vi "Next.vi"(0 "object in":refnum<class "BFSTreeIterator.lvclass">, 5 "Error In":errorcluster) -> (14 "object out":refnum<class "BFSTreeIterator.lvclass">, 16 "Next":refnum<class "Element.lvclass">, 19 "Error Out":errorcluster)   [LabVIEW 2024, in "BFSTreeIterator.lvclass"]
doc: "Gets next item in the traversal order. Also prepare for upcoming nodes."
uses:
  BFSTreeIterator.lvclass
  Element_interface/Element.lvclass
  BFSTreeIterator.lvclass/BFSTreeIterator.ctl
  Node_class/Node.lvclass
  C:/Users/burakkorkmaz/Desktop/Leveling/labview-desing-patterns/Iterator Pattern/Element_interface/Element.lvclass
panel:
  # "Connector Pane"
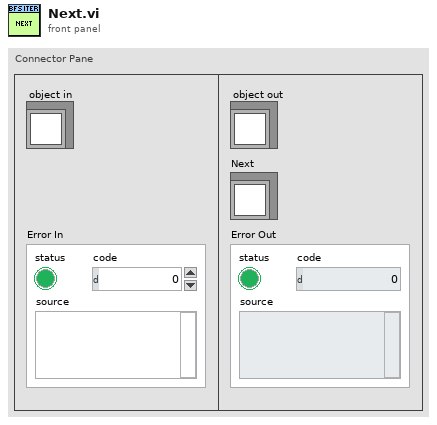
[diagram p1: front panel]
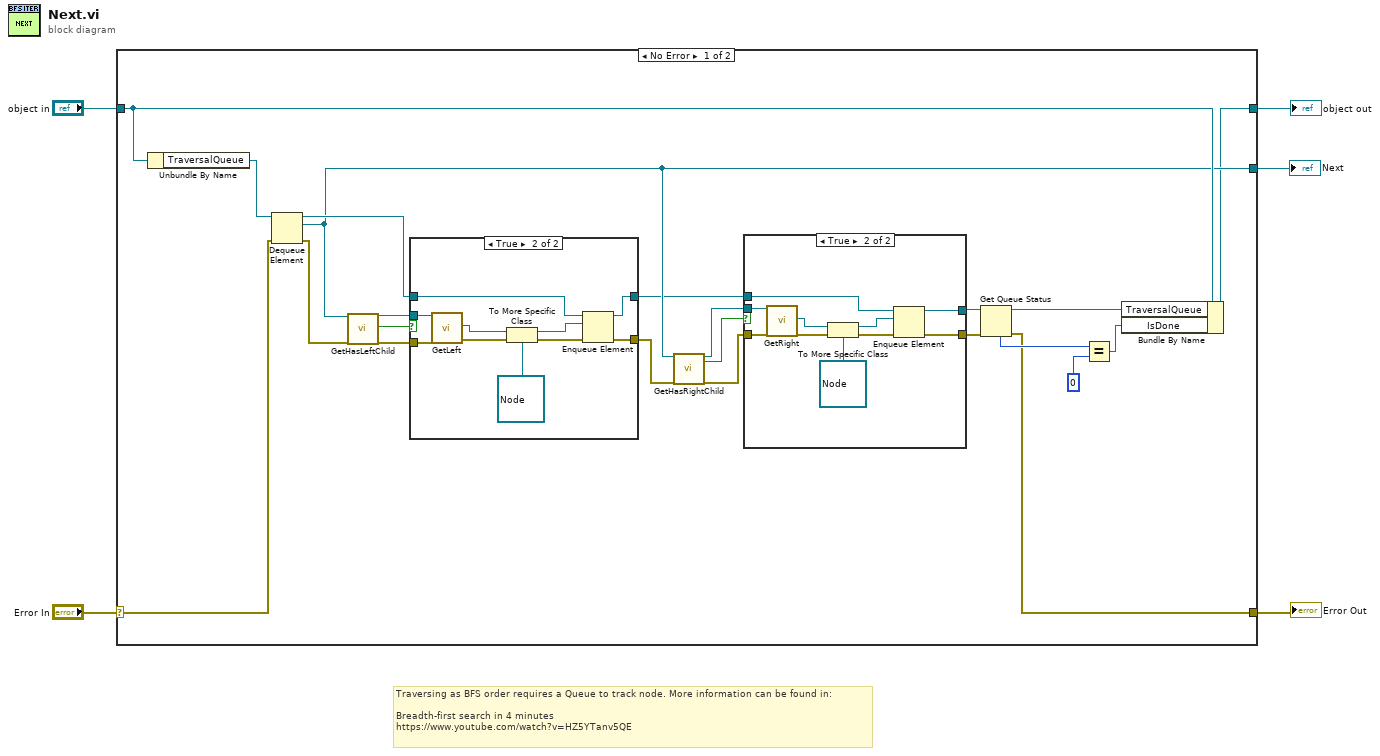
[diagram p0: block diagram]
diagram:
  # "Traversing as BFS order requires a Queue to track node. More information can be found in:\n\nBreadth-first search in 4 minutes\nhttps://www.youtube.com/watch?v=HZ5YTanv5QE"
  n1 = case shown="No Error" "Error In" {
    selector: "Error In" -> [w25 w53]
    tunnel: [w6 w53] -> w4
    tunnel: [w13 w52] -> w2
    tunnel: "object in" -> [w27 w52]
    tunnel: [w19 _] -> w1
    frame No Error {
      n2 = Unbundle By Name(w27) -> ("TraversalQueue"=w26:refnum<queue>)
      n3 = Dequeue Element(queue=w26, error in (no error)=w25) -> (queue out=w20:refnum<queue>, element=w19:refnum<class "Node.lvclass">, error out=w23:errorcluster)  [unwired: 1 in, 1 out]
      n4 = call-dynamic "GetHasLeftChild.vi"("object in"=w19, "Error In"=w23) -> ("object out"=w22:refnum<class "Node.lvclass">, "HasLeftChild"=w24:bool, "Error Out"=w21:errorcluster)  [unwired: 15 in]
      n5 = case shown="True" w24 {
        tunnel: w22 -> [_ w51]
        tunnel: w21 -> [w41 w50]
        tunnel: w20 -> [w40 w49]
        tunnel: [w40 w42] -> w14
        tunnel: [w41 w43] -> w18
        frame False {
        }
        frame True {
          n6 = call-dynamic "GetLeft.vi"("object in"=w51, "Error In"=w50) -> ("Left"=w46:refnum<class "Element.lvclass">, "Error Out"=w48:errorcluster)  [unwired: 15 in, 1 out]
          n7 = To More Specific Class(target class=refnum<class "Node.lvclass"> refnum ("Node"), reference=w46, error in=w48) -> (specific class reference=w45:refnum<class "Node.lvclass">, error out=w47:errorcluster)
          n8 = Enqueue Element(queue=w49, element=w45, error in (no error)=w47) -> (queue out=w42:refnum<queue>, error out=w43:errorcluster)  [unwired: 1 in, 1 out]
        }
      }
      n9 = call-dynamic "GetHasRightChild.vi"("object in"=w19, "Error In"=w18) -> ("object out"=w16:refnum<class "Node.lvclass">, "HasRightChild"=w17:bool, "Error Out"=w15:errorcluster)  [unwired: 15 in]
      n10 = case shown="True" w17 {
        tunnel: w16 -> [_ w38]
        tunnel: w15 -> [w28 w39]
        tunnel: [w29 w32] -> w11
        tunnel: [w28 w31] -> w12
        tunnel: w14 -> [w29 w30]
        frame False {
        }
        frame True {
          n11 = call-dynamic "GetRight.vi"("object in"=w38, "Error In"=w39) -> ("Right"=w37:refnum<class "Element.lvclass">, "Error Out"=w36:errorcluster)  [unwired: 15 in, 1 out]
          n12 = To More Specific Class(target class=refnum<class "Node.lvclass"> refnum ("Node"), reference=w37, error in=w36) -> (specific class reference=w34:refnum<class "Node.lvclass">, error out=w35:errorcluster)
          n13 = Enqueue Element(queue=w30, element=w34, error in (no error)=w35) -> (queue out=w32:refnum<queue>, error out=w31:errorcluster)  [unwired: 1 in, 1 out]
        }
      }
      n14 = Get Queue Status(queue=w11, error in (no error)=w12) -> (queue out=w7:refnum<queue>, error out=w6:errorcluster, # elements in queue=w10:i32)  [unwired: 1 in, 5 out]
      n15 = Equal?(x=w10, y=0) -> (x = y?=w8:bool)
      n16 = Bundle By Name(cluster=w27, "TraversalQueue"=w7, "IsDone"=w8) -> (w13:refnum<class "BFSTreeIterator.lvclass">)
    }
    frame Error {
    }
  }
  "Error Out" <- w4
  "object out" <- w2
  "Next" <- w1
